vi "setName.vi"(0 "reference":refnum<class "ImplicitParameterNode.lvclass">, 1 "name":refnum<class "MultiLineString.lvclass">, 5 "error in (no error)":errorcluster) -> (14 "reference out":refnum<class "ImplicitParameterNode.lvclass">, 19 "error out":errorcluster)   [LabVIEW 2016, in "ImplicitParameterNode.lvclass"]
doc: "public void setName(MultiLineString n)"
uses:
  <resource>/Framework/Providers/Open_GDS/UML/ImplicitParameterNode_class/ImplicitParameterNode.lvclass
  <resource>/Framework/Providers/Open_GDS/UML/MultiLineString_class/MultiLineString.lvclass
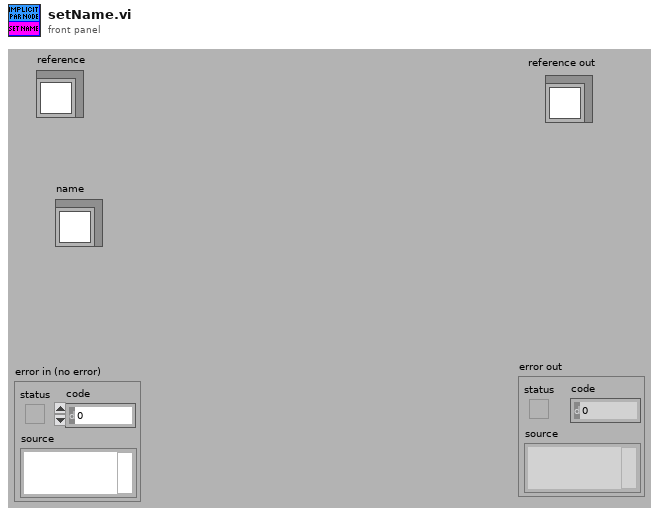
[diagram p1: front panel]
types:
  T1 = typedef "ImplicitParameterNode.lvclass/ObjectAttributes.ctl" = cluster{"topHeight":dbl, "name":refnum<class "MultiLineString.lvclass">, "DEFAULT_TOP_HEIGHT":i32, "DEFAULT_WIDTH":i32, "DEFAULT_HEIGHT":i32}
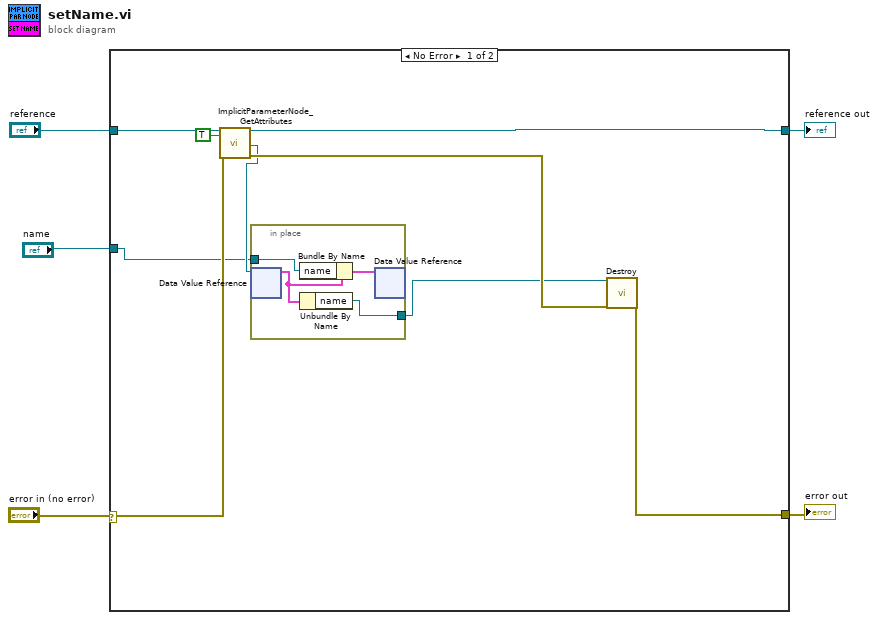
[diagram p0: block diagram]
diagram:
  n1 = case shown="No Error" "error in (no error)" {
    selector: "error in (no error)" -> [w11 w19]
    tunnel: "reference" -> [w14 w20]
    tunnel: [w13 w19] -> w4
    tunnel: [w12 w20] -> w3
    tunnel: "name" -> [w7 _]
    frame No Error {
      n2 = call <resource>:"ImplicitParameterNode_GetAttributes.vi"("reference in"=w14, "OnlyGetDvrReference(False)"=TRUE, "error in (no error)"=w11) -> ("reference out"=w12:refnum<class "ImplicitParameterNode.lvclass">, "DataRef"=w8:refnum<data-value>, "error out"=w10:errorcluster)  [unwired: 13 in, 1 out]
      n3 = in-place {
        in-place-border: w7 -> [w17]
        in-place-border: [w15] -> w6
        n4 = in-place-dvr #1(w8) -> (w18:T1)  [unwired: 1 out]
        n5 = Bundle By Name(cluster=w18, "name"=w17) -> (w16:T1)
        n6 = Unbundle By Name(w18) -> ("name"=w15:refnum<class "MultiLineString.lvclass">)
        n7 = in-place-dvr #1(w16) -> ()  [unwired: 2 out]
      }
      n8 = call-dynamic "Destroy.vi"("reference"=w6, "error in (no error)"=w10) -> ("error out"=w13:errorcluster)  [unwired: 17 out]
    }
    frame Error {
    }
  }
  "reference out" <- w3
  "error out" <- w4
